vi "save configuration.vi"(10 "Waveform chart":refnum<vi>, 11 "selected parameters":string[](array[string])) -> ()   [LabVIEW 2016]
uses:
  configuration file type def.ctl
  Communication Global variables.vi
  <vilib>/addons/_JKI.lib/Serialization/JSON/JKI JSON Serialization.lvlib
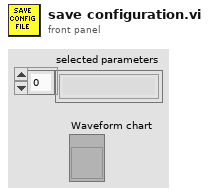
[diagram p1: front panel]
types:
  T1 = typedef "configuration file type def.ctl" = cluster{"selected parameters":string[], "REST URL":string, "UDP port":u16, "XScale.Minimum":dbl, "XScale.Maximum":dbl, "Yscale mins":dbl[], "Yscale maxs":dbl[], "Yscale colors":u32[], "LegNumRows":u32, "plot colors":u32[], "plot pointstyles":u8[], "plot names":string[], "plot yscale selections":u32[], "plot visibles":bool[]}
  T2 = enum16{"open", "replace", "create", "open or create", "replace or create", "replace or create with confirmation"}
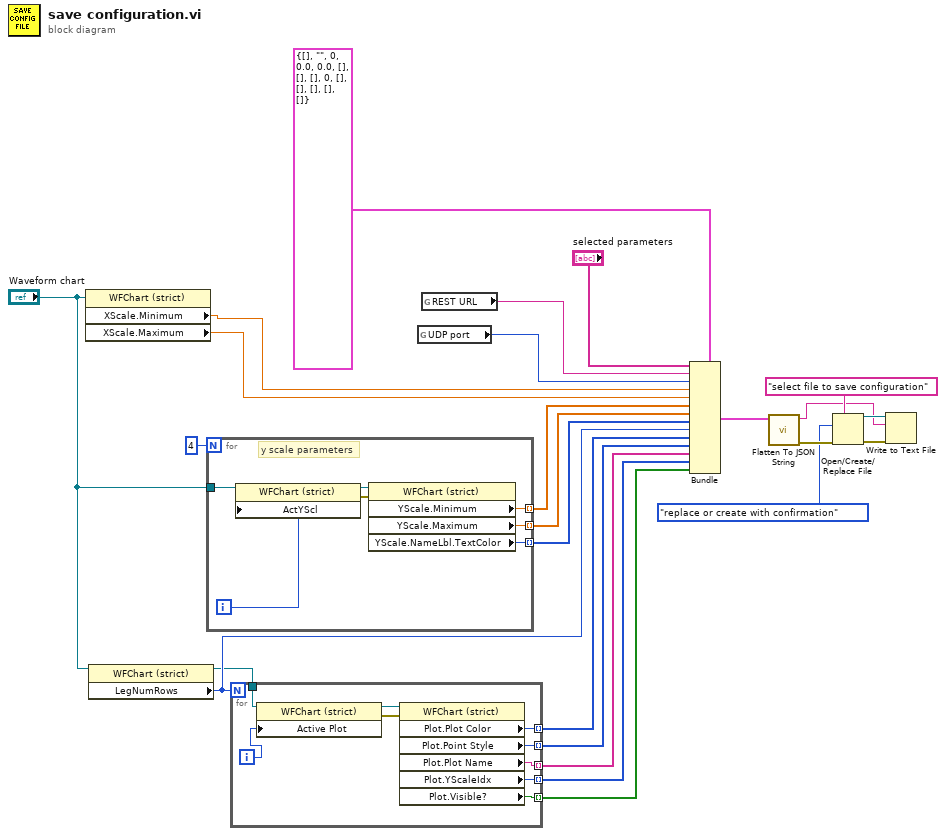
[diagram p0: block diagram]
diagram:
  n1 = property class="WFChart (strict)"(reference="Waveform chart") -> ("XScale.Minimum"=w22:dbl, "XScale.Maximum"=w21:dbl)  [unwired: 1 in, 2 out]
  n2 = property class="WFChart (strict)"(reference="Waveform chart") -> (reference out=w5:refnum<vi>, "LegNumRows"=w16:u32)  [unwired: 1 in, 1 out]
  n3 = for {
    N: 4 -> [_]
    tunnel: "Waveform chart" -> [w31]
    tunnel: [w28] -> w20 mode=indexing
    tunnel: [w27] -> w19 mode=indexing
    tunnel: [w26] -> w18 mode=indexing
    i -> [w32]
    # "y scale parameters"
    n4 = property class="WFChart (strict)"(reference=w31, "ActYScl"=w32) -> (reference out=w30:refnum<vi>, error out=w29:errorcluster)  [unwired: 1 in]
    n5 = property class="WFChart (strict)"(reference=w30, error in=w29) -> ("YScale.Minimum"=w28:dbl, "YScale.Maximum"=w27:dbl, "YScale.NameLbl.TextColor"=w26:u32)  [unwired: 2 out]
  }
  n6 = for {
    N: w16 -> [_]
    tunnel: [w38] -> w15 mode=indexing
    tunnel: [w37] -> w14 mode=indexing
    tunnel: [w36] -> w13 mode=indexing
    tunnel: [w35] -> w12 mode=indexing
    tunnel: [w34] -> w11 mode=indexing
    tunnel: w5 -> [w33]
    i -> [w41]
    n7 = property class="WFChart (strict)"(reference=w33, "Active Plot"=w41) -> (reference out=w39:refnum<vi>, error out=w40:errorcluster)  [unwired: 1 in]
    n8 = property class="WFChart (strict)"(reference=w39, error in=w40) -> ("Plot.Plot Color"=w38:u32, "Plot.Point Style"=w37:u8, "Plot.Plot Name"=w36:string, "Plot.YScaleIdx"=w35:u32, "Plot.Visible?"=w34:bool)  [unwired: 2 out]
  }
  n9 = global read "Communication Global variables.vi" "UDP port"() -> (w2:u16)
  n10 = global read "Communication Global variables.vi" "REST URL"() -> (w3:string)
  n11 = Bundle(cluster=T1 {"selected parameters"=[], "REST URL"="", "UDP port"=0, "XScale.Minimum"=0.0, "XScale.Maximum"=0.0, "Yscale mins"=[], "Yscale maxs"=[], "Yscale colors"=[], "LegNumRows"=0, "plot colors"=[], "plot pointstyles"=[], "plot names"=[], "plot yscale selections"=[], "plot visibles"=[]} ("output cluster"), "selected parameters"="selected parameters", "REST URL"=w3, "UDP port"=w2, "XScale.Minimum"=w22, "XScale.Maximum"=w21, "Yscale mins"=w20, "Yscale maxs"=w19, "Yscale colors"=w18, "LegNumRows"=w16, "plot colors"=w15, "plot pointstyles"=w14, "plot names"=w13, "plot yscale selections"=w12, "plot visibles"=w11) -> (w10:T1)
  n12 = call <vilib>:"Flatten To JSON String.vi"("Variant"=w10) -> ("error out"=w9:errorcluster, "JSON String"=w6:string)  [unwired: 9 in]
  n13 = Open/Create/Replace File(error in=w9, prompt="select file to save configuration", operation (0:open)=T2."replace or create with confirmation") -> (refnum out=w7:refnum<file>, error out=w8:errorcluster)  [unwired: 3 in, 1 out]
  n14 = Write to Text File(file (use dialog)=w7, text=w6, error in=w8) -> ()  [unwired: 1 in, 3 out]
